vi "Polynomial Interpolation.vi"(3 "x value":dbl format="%0.2f", 4 "X":dbl[](array[numeric]) format="%0.2f", 5 "Y":dbl[](array[numeric]) format="%0.2f") -> (0 "error":i32, 1 "interpolation error":dbl format="%0.2f", 2 "interpolation value":dbl format="%0.2f")   [LabVIEW 2024, in "NI_AALPro.lvlib"]
doc: "<p>Interpolates or extrapolates the function f at x given a set of n points (x[i]y[i]), where f(x[i]) = y[i], f is any function, and given a number <strong>x value</strong>.</p>"
uses:
  NI_AALPro.lvlib
  <resource>/lvanlys.dll
panel:
  # "Polynomial Interpolation"
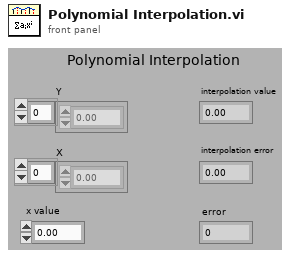
[diagram p1: front panel]
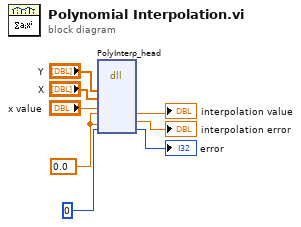
[diagram p0: block diagram]
diagram:
  w5 = 0.0
  n1 = dll-call lib="C:/Program Files (x86)/National Instruments/LabVIEW 2024/resource/lvanlys.*" fn="PolyInterp_head"("Y"="Y", "X"="X", "x value"="x value", "output param"=w5, "output param"=w5, "output param"=0) -> ("output param"=→"interpolation value":dbl, "output param"=→"interpolation error":dbl, "output param"=→"error":i32)  [unwired: 7 in, 2 out]
